vi "MakeSnakeFat.vi"(11 "line_hor":u16) -> (3 "Numeric":u16)   [LabVIEW 2019, in "RT_Game.lvlib" / "Snake.lvclass"]
uses:
  Snake.lvclass
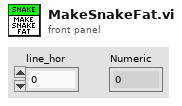
[diagram p1: front panel]
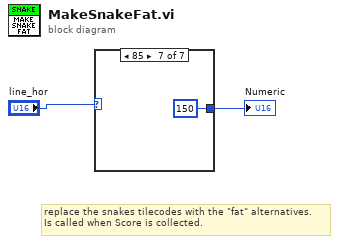
[diagram p0: block diagram]
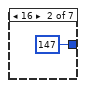
[diagram p3: hidden frame]
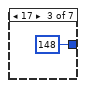
[diagram p4: hidden frame]
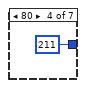
[diagram p5: hidden frame]
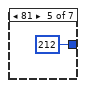
[diagram p6: hidden frame]
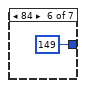
[diagram p7: hidden frame]
diagram:
  # "replace the snakes tilecodes with the \"fat\" alternatives.\nIs called when Score is collected."
  n1 = case shown="85" "line_hor" {
    selector: "line_hor" -> [w3 _ _ _ _ _ _]
    tunnel: [w3 u16 147 ("line_hor") u16 148 ("line_hor") u16 211 ("line_hor") u16 212 ("line_hor") u16 149 ("line_hor") u16 150 ("line_hor")] -> w1
    frame 0, Default {
    }
    frame 16 {
    }
    frame 17 {
    }
    frame 80 {
    }
    frame 81 {
    }
    frame 84 {
    }
    frame 85 {
    }
  }
  "Numeric" <- w1
